vi "Control - Direct Injection.vi"(0 "Fuel Desired [mg/cyc]":sgl, 5 "MEP Desired [bar]":sgl, 11 "Control Inputs":T3={"Engine Speed [RPM]"=0.0, "Engine Status"=enum."STALLED", "Load Control \nMode"=enum."Max Speed Governor", "dt(s)"=0.0, "Number of Cylinders"=0, "Engine Displacement [cc]"=0.0, "StoichAFR"=0.0, "Q.LHV Fuel [kJ/kg]"=0.0, "BattV PSU [V]"=0.0, "12V PSU [V]"=0.0, "5V PSU [V]"=0.0, "Pedal Position [%]"=0.0, "Oil Pressure [kPa]"=0.0, "Oil Temp [C]"=0.0, "Oil Level [%]"=0.0, "Engine Coolant Temp (ECT) [C]"=0.0, "Engine Coolant Pressure [kPa]"=0.0, "Rail Pressure [bar]"=0.0, "Fuel Pressure [kPa]"=0.0, "Fuel Temp [C]"=0.0, "Vacuum Pressure [kPa]"=0.0, "Throttle Position [%]"=0.0, "Cam1 Advance [CAD]"=0.0, "Cam2 Advance [CAD]"=0.0, "Cam3 Advance [CAD]"=0.0, "Cam4 Advance [CAD]"=0.0, "CA50 Control Output [CAD]"=[], "CA50 Control Output Valid"=[], "Intake Air Temp (IAT) [C]"=0.0, "Barometric Air Pressure [kPa]"=0.0, "Intake Air Rel. Humidity [%]"=0.0, "Mass Air Flow (MAF) [kg/hr]"=0.0, "Turbo Inlet Air Pressure [kPa]"=0.0, "Turbo Inlet Air Temp [C]"=0.0, "Turbo Outlet Air Pressure [kPa]"=0.0, "Turbo Outlet Air Temp [C]"=0.0, "CAC Outlet Pressure [kPa]"=0.0, "CAC Outlet Temp [C]"=0.0, "Intake Manifold Pressure (MAP) [kPa]"=0.0, "Intake Manifold Temp (MAT) [C]"=0.0, "Exhaust Manifold Pressure [kPa]"=0.0, "Exhaust Manifold Temp [C]"=0.0, "HighP EGR Cooler Outlet Pressure [kPa]"=0.0, "HighP EGR Cooler Outlet Temp [C]"=0.0, "HighP EGR Differential Pressure [kPa]"=0.0, "HighP EGR Valve Position [%]"=0.0, "Turbo Outlet Exhaust Pressure [kPa]"=0.0, "Turbo Outlet Exhaust Temp [C]"=0.0, "VGT Position 1 [%]"=0.0, "VGT Position 2 [%]"=0.0, "Turbo Speed 1 [RPM]"=0.0, "Turbo Speed 2 [RPM]"=0.0, "LowP EGR Differential Pressure [kPa]"=0.0, "LowP EGR Valve Position [%]"=0.0, "UEGO1Lambda"=0.0, "UEGO1_Hot"=FALSE, "UEGO2Lambda"=0.0, "UEGO2_Hot"=FALSE, "Knock Intensity"=[], "Knock"=[]} {"Knock Intensity" format="%.2f"; "CA50 Control Output [CAD]" format="%.2f"; "Exhaust Manifold Temp [C]" format="%#_6f"; "UEGO2Lambda" format="%.2f"; "Intake Manifold Temp (MAT) [C]" format="%#_6f"; "UEGO1Lambda" format="%.2f"}) -> (4 "DI Quantities Desired [mg/inj]":T2[](array[typedef]), 8 "DI Timings Desired [DBTDC]":T1[](array[typedef]))   [LabVIEW 2015, in "ECS-RT.lvlib"]
uses:
  ECS-RT.lvlib
  Typedefs/Control Inputs/Control Inputs.ctl
  Typedefs/EPT/Engine Status.ctl
  Typedefs/MISC/Load Control Mode.ctl
  Typedefs/Control Outputs/Injection Quantity.ctl
  Typedefs/Control Outputs/Injection Timing.ctl
  ECS-Shared.lvlib
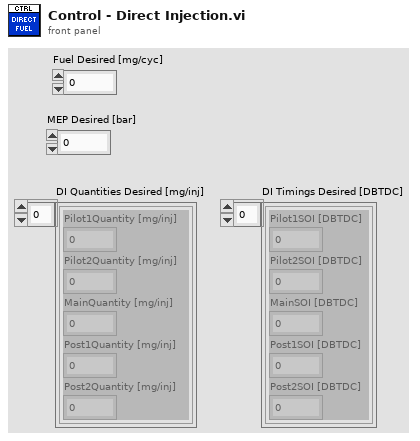
[diagram p1: front panel]
types:
  T1 = typedef "ECS-Shared.lvlib/Injection Timing.ctl" = cluster{"Pilot1SOI [DBTDC]":sgl, "Pilot2SOI [DBTDC]":sgl, "MainSOI [DBTDC]":sgl, "Post1SOI [DBTDC]":sgl, "Post2SOI [DBTDC]":sgl}
  T2 = typedef "ECS-Shared.lvlib/Injection Quantity.ctl" = cluster{"Pilot1Quantity [mg/inj]":sgl, "Pilot2Quantity [mg/inj]":sgl, "MainQuantity [mg/inj]":sgl, "Post1Quantity [mg/inj]":sgl, "Post2Quantity [mg/inj]":sgl}
  T3 = typedef "ECS-Shared.lvlib/Control Inputs.ctl" = cluster{"Engine Speed [RPM]":sgl, "Engine Status":T4, "Load Control \nMode":T5, "dt(s)":sgl, "Number of Cylinders":u8, "Engine Displacement [cc]":sgl, "StoichAFR":sgl, "Q.LHV Fuel [kJ/kg]":sgl, "BattV PSU [V]":sgl, "12V PSU [V]":sgl, "5V PSU [V]":sgl, "Pedal Position [%]":sgl, "Oil Pressure [kPa]":sgl, "Oil Temp [C]":sgl, "Oil Level [%]":sgl, "Engine Coolant Temp (ECT) [C]":sgl, "Engine Coolant Pressure [kPa]":sgl, "Rail Pressure [bar]":sgl, "Fuel Pressure [kPa]":sgl, "Fuel Temp [C]":sgl, "Vacuum Pressure [kPa]":sgl, "Throttle Position [%]":sgl, "Cam1 Advance [CAD]":sgl, "Cam2 Advance [CAD]":sgl, "Cam3 Advance [CAD]":sgl, "Cam4 Advance [CAD]":sgl, "CA50 Control Output [CAD]":sgl[], "CA50 Control Output Valid":bool[], "Intake Air Temp (IAT) [C]":sgl, "Barometric Air Pressure [kPa]":sgl, "Intake Air Rel. Humidity [%]":sgl, "Mass Air Flow (MAF) [kg/hr]":sgl, "Turbo Inlet Air Pressure [kPa]":sgl, "Turbo Inlet Air Temp [C]":sgl, "Turbo Outlet Air Pressure [kPa]":sgl, "Turbo Outlet Air Temp [C]":sgl, "CAC Outlet Pressure [kPa]":sgl, "CAC Outlet Temp [C]":sgl, "Intake Manifold Pressure (MAP) [kPa]":sgl, "Intake Manifold Temp (MAT) [C]":sgl, "Exhaust Manifold Pressure [kPa]":sgl, "Exhaust Manifold Temp [C]":sgl, "HighP EGR Cooler Outlet Pressure [kPa]":sgl, "HighP EGR Cooler Outlet Temp [C]":sgl, "HighP EGR Differential Pressure [kPa]":sgl, "HighP EGR Valve Position [%]":sgl, "Turbo Outlet Exhaust Pressure [kPa]":sgl, "Turbo Outlet Exhaust Temp [C]":sgl, "VGT Position 1 [%]":sgl, "VGT Position 2 [%]":sgl, "Turbo Speed 1 [RPM]":sgl, "Turbo Speed 2 [RPM]":sgl, "LowP EGR Differential Pressure [kPa]":sgl, "LowP EGR Valve Position [%]":sgl, "UEGO1Lambda":sgl, "UEGO1_Hot":bool, "UEGO2Lambda":sgl, "UEGO2_Hot":bool, "Knock Intensity":sgl[], "Knock":bool[]}
  T4 = typedef "ECS-Shared.lvlib/Engine Status.ctl" = enum16{"OFF", "STALLED", "CRANKING", "RUNNING", "ACCEL", "DECEL", "SAFE"}
  T5 = typedef "ECS-Shared.lvlib/Load Control Mode.ctl" = enum16{"No Governor", "Min Speed Governor", "Max Speed Governor"}
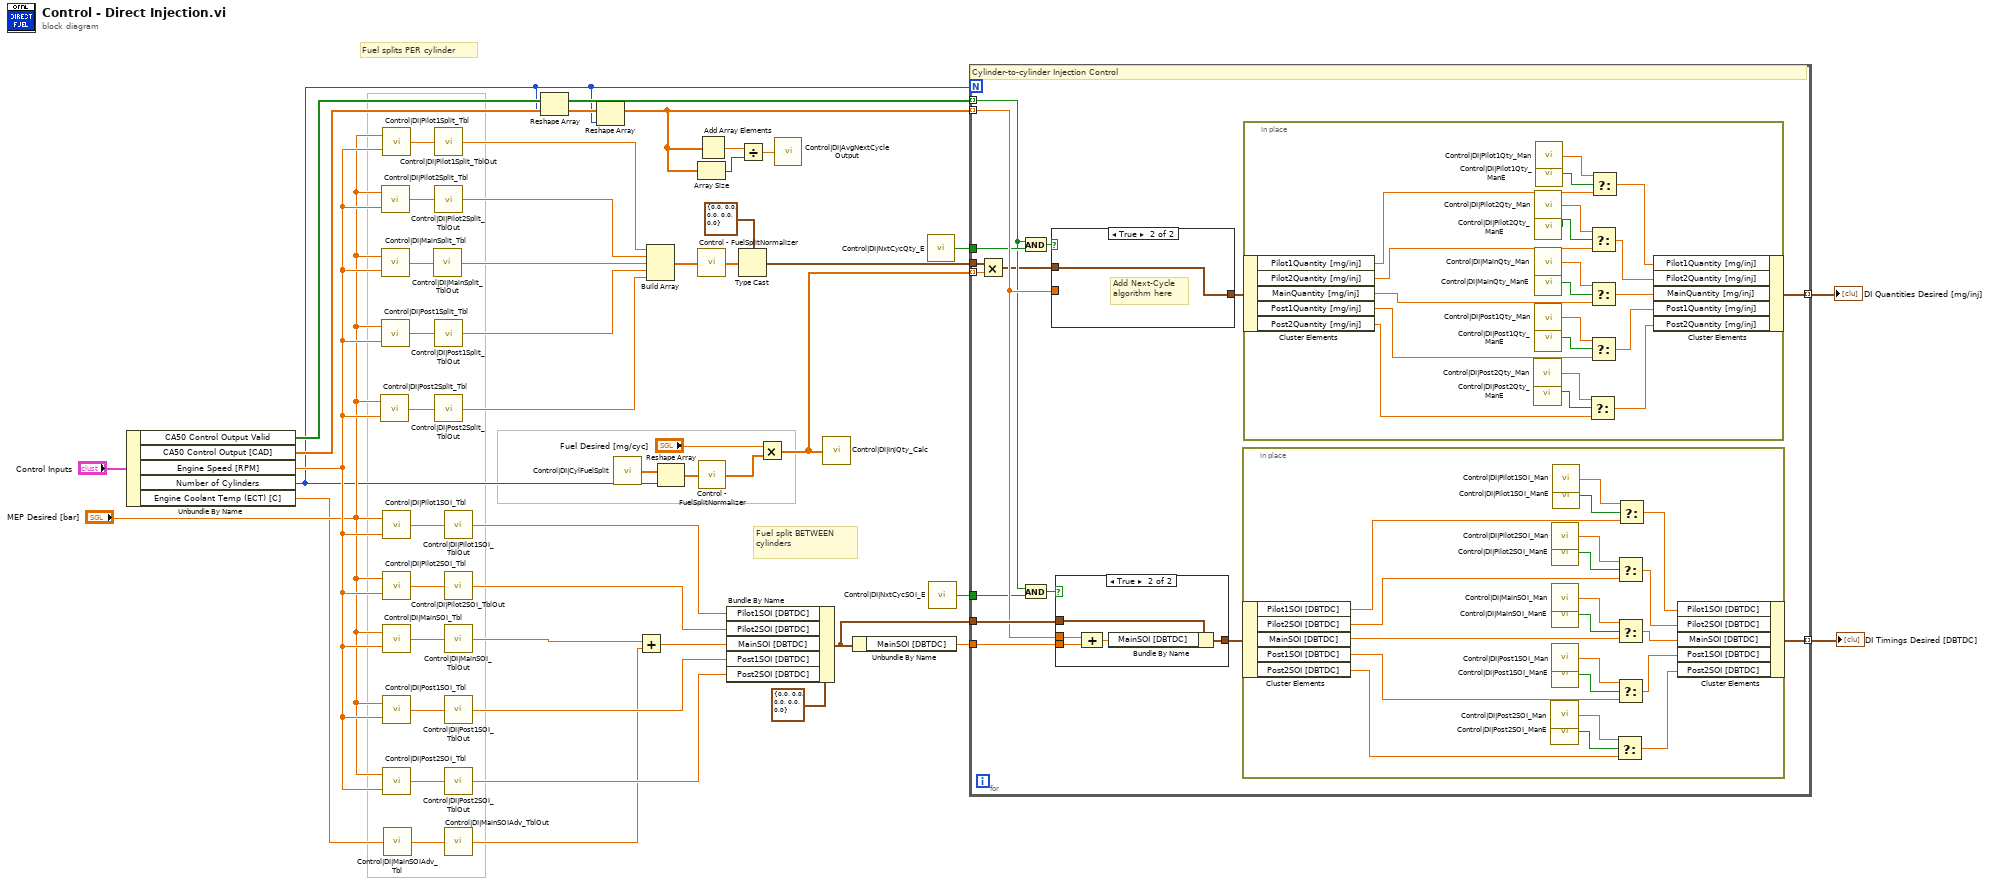
[diagram p0: block diagram]
diagram:
  # "Fuel split BETWEEN cylinders"
  # "Fuel splits PER cylinder"
  n1 = Unbundle By Name("Control Inputs") -> ("CA50 Control Output Valid"=w4:bool[], "CA50 Control Output [CAD]"=w5:sgl[], "Engine Speed [RPM]"=w20:sgl, "Number of Cylinders"=w1:u8, "Engine Coolant Temp (ECT) [C]"=w11:sgl)
  n2 = call "Control|DI|Post2Split_Tbl"("Y Index"=w20, "X Index"="MEP Desired [bar]") -> ("Z"=w29:sgl)
  n3 = call "Control|DI|Pilot2Split_Tbl"("Y Index"=w20, "X Index"="MEP Desired [bar]") -> ("Z"=w32:sgl)
  n4 = call "Control|DI|MainSplit_Tbl"("Y Index"=w20, "X Index"="MEP Desired [bar]") -> ("Z"=w31:sgl)
  n5 = call "Control|DI|Post1Split_Tbl"("Y Index"=w20, "X Index"="MEP Desired [bar]") -> ("Z"=w30:sgl)
  n6 = call "Control|DI|Pilot1Split_Tbl"("Y Index"=w20, "X Index"="MEP Desired [bar]") -> ("Z"=w33:sgl)
  n7 = call "Control|DI|Pilot1SOI_Tbl"("Y Index"=w20, "X Index"="MEP Desired [bar]") -> ("Z"=w40:sgl)
  n8 = call "Control|DI|Pilot2SOI_Tbl"("Y Index"=w20, "X Index"="MEP Desired [bar]") -> ("Z"=w39:sgl)
  n9 = call "Control|DI|MainSOI_Tbl"("Y Index"=w20, "X Index"="MEP Desired [bar]") -> ("Z"=w17:sgl)
  n10 = call "Control|DI|Post1SOI_Tbl"("Y Index"=w20, "X Index"="MEP Desired [bar]") -> ("Z"=w38:sgl)
  n11 = call "Control|DI|Post2SOI_Tbl"("Y Index"=w20, "X Index"="MEP Desired [bar]") -> ("Z"=w37:sgl)
  n12 = call "Control|DI|MainSOIAdv_Tbl"("X Index"=w11) -> ("Y"=w15:sgl)
  n13 = call "Control|DI|MainSplit_TblOut"("Value"=w31) -> ()
  n14 = call "Control|DI|Pilot1Split_TblOut"("Value"=w33) -> ()
  n15 = call "Control|DI|Pilot2Split_TblOut"("Value"=w32) -> ()
  n16 = call "Control|DI|Post1Split_TblOut"("Value"=w30) -> ()
  n17 = call "Control|DI|Post2Split_TblOut"("Value"=w29) -> ()
  n18 = call "Control|DI|Pilot1SOI_TblOut"("Value"=w40) -> ()
  n19 = call "Control|DI|Pilot2SOI_TblOut"("Value"=w39) -> ()
  n20 = call "Control|DI|MainSOI_TblOut"("Value"=w17) -> ()
  n21 = call "Control|DI|Post1SOI_TblOut"("Value"=w38) -> ()
  n22 = call "Control|DI|Post2SOI_TblOut"("Value"=w37) -> ()
  n23 = call "Control|DI|MainSOIAdv_TblOut"("Value"=w15) -> ()
  n24 = Reshape Array(w4, w1) -> (w2:bool[])
  n25 = Reshape Array(w5, w1) -> (w3:sgl[])
  n26 = call "Control|DI|CylFuelSplit"() -> ("Value"=w10:sgl[])
  n27 = Add(x=w17, y=w15) -> (x+y=w16:sgl)
  n28 = Build Array(w33, w32, w31, w30, w29) -> (w28:sgl[])
  n29 = Reshape Array(w10, w1) -> (w9:sgl[])
  n30 = Array Size(array=w3) -> (size(s)=w26:i32)
  n31 = call "Control - FuelSplitNormalizer.vi"("Fuel Splits []"=w28) -> ("Normalized Fuel Splits [Frac]"=w7:sgl[])  [unwired: 14 in]
  n32 = call "Control - FuelSplitNormalizer.vi"("Fuel Splits []"=w9) -> ("Normalized Fuel Splits [Frac]"=w14:sgl[])  [unwired: 14 in]
  n33 = Add Array Elements(numeric array=w3) -> (sum=w27:sgl)
  n34 = Bundle By Name(cluster=T1 {"Pilot1SOI [DBTDC]"=0.0, "Pilot2SOI [DBTDC]"=0.0, "MainSOI [DBTDC]"=0.0, "Post1SOI [DBTDC]"=0.0, "Post2SOI [DBTDC]"=0.0} ("FuelTiming [DBTDC] 2"), "Pilot1SOI [DBTDC]"=w40, "Pilot2SOI [DBTDC]"=w39, "MainSOI [DBTDC]"=w16, "Post1SOI [DBTDC]"=w38, "Post2SOI [DBTDC]"=w37) -> (w36:T1)
  n35 = Type Cast(type=T2 {"Pilot1Quantity [mg/inj]"=0.0, "Pilot2Quantity [mg/inj]"=0.0, "MainQuantity [mg/inj]"=0.0, "Post1Quantity [mg/inj]"=0.0, "Post2Quantity [mg/inj]"=0.0} ("Injection Quantity [mg/inj]"), x=w7) -> (*(type *) &x=w6:T2)
  n36 = Divide(x=w27, y=w26) -> (x/y=w25:sgl)
  n37 = Multiply(x="Fuel Desired [mg/cyc]", y=w14) -> (x*y=w13:sgl[])
  n38 = call "Control|DI|AvgNextCycleOutput"("Value"=w25) -> ()
  n39 = call "Control|DI|InjQty_Calc"("Value"=w13) -> ()
  n40 = Unbundle By Name(w36) -> ("MainSOI [DBTDC]"=w23:sgl)
  n41 = call "Control|DI|NxtCycQty_E"() -> ("Value"=w21:bool)
  n42 = call "Control|DI|NxtCycSOI_E"() -> ("Value"=w24:bool)
  n43 = for {
    N: w1 -> [_]
    tunnel: [w53] -> w34 mode=indexing
    tunnel: w23 -> [w49]
    tunnel: w36 -> [w55]
    tunnel: w24 -> [w44]
    tunnel: [w51] -> w22 mode=indexing
    tunnel: w2 -> [w45] mode=indexing
    tunnel: w3 -> [w48] mode=indexing
    tunnel: w21 -> [w46]
    tunnel: w6 -> [w42]
    tunnel: w13 -> [w43] mode=indexing
    # "Cylinder-to-cylinder Injection Control"
    n44 = Multiply(x=w42, y=w43) -> (x*y=w41:T2)
    n45 = And(x=w45, y=w46) -> (x .and. y?=w47:bool)
    n46 = And(x=w45, y=w44) -> (x .and. y?=w52:bool)
    n47 = case shown="True" w47 {
      tunnel: w48 -> [_ _]
      tunnel: [w56 w57] -> w50
      tunnel: w41 -> [w56 w57]
      frame False {
      }
      frame True {
        # "Add Next-Cycle\nalgorithm here"
      }
    }
    n48 = case shown="True" w52 {
      tunnel: [w98 w102] -> w54
      tunnel: w55 -> [w98 w99]
      tunnel: w49 -> [_ w101]
      tunnel: w48 -> [_ w100]
      frame False {
      }
      frame True {
        n49 = Compound Arithmetic op=ADD(w100, w101) -> (w103:sgl)
        n50 = Bundle By Name(cluster=w99, "MainSOI [DBTDC]"=w103) -> (w102:T1)
      }
    }
    n51 = in-place {
      n52 = in-place-cluster #1(w54) -> ("Pilot1SOI [DBTDC]"=w87:sgl, "Pilot2SOI [DBTDC]"=w86:sgl, "MainSOI [DBTDC]"=w85:sgl, "Post1SOI [DBTDC]"=w84:sgl, "Post2SOI [DBTDC]"=w83:sgl)
      n53 = call "Control|DI|Post2SOI_Man"() -> ("Value"=w96:sgl)
      n54 = call "Control|DI|Post2SOI_ManE"() -> ("Value"=w97:bool)
      n55 = call "Control|DI|Pilot2SOI_Man"() -> ("Value"=w92:sgl)
      n56 = call "Control|DI|Pilot2SOI_ManE"() -> ("Value"=w93:bool)
      n57 = call "Control|DI|MainSOI_Man"() -> ("Value"=w88:sgl)
      n58 = call "Control|DI|MainSOI_ManE"() -> ("Value"=w89:bool)
      n59 = call "Control|DI|Post1SOI_Man"() -> ("Value"=w94:sgl)
      n60 = call "Control|DI|Post1SOI_ManE"() -> ("Value"=w95:bool)
      n61 = call "Control|DI|Pilot1SOI_Man"() -> ("Value"=w90:sgl)
      n62 = call "Control|DI|Pilot1SOI_ManE"() -> ("Value"=w91:bool)
      n63 = Select(t=w96, s=w97, f=w83) -> (s? t:f=w78:sgl)
      n64 = Select(t=w92, s=w93, f=w86) -> (s? t:f=w81:sgl)
      n65 = Select(t=w88, s=w89, f=w85) -> (s? t:f=w80:sgl)
      n66 = Select(t=w94, s=w95, f=w84) -> (s? t:f=w79:sgl)
      n67 = Select(t=w90, s=w91, f=w87) -> (s? t:f=w82:sgl)
      n68 = in-place-cluster #1("Pilot1SOI [DBTDC]"=w82, "Pilot2SOI [DBTDC]"=w81, "MainSOI [DBTDC]"=w80, "Post1SOI [DBTDC]"=w79, "Post2SOI [DBTDC]"=w78) -> (w53:T1)
    }
    n69 = in-place {
      n70 = in-place-cluster #2(w50) -> ("Pilot1Quantity [mg/inj]"=w62:sgl, "Pilot2Quantity [mg/inj]"=w61:sgl, "MainQuantity [mg/inj]"=w60:sgl, "Post1Quantity [mg/inj]"=w59:sgl, "Post2Quantity [mg/inj]"=w58:sgl)
      n71 = call "Control|DI|Post2Qty_Man"() -> ("Value"=w69:sgl)
      n72 = call "Control|DI|Post2Qty_ManE"() -> ("Value"=w68:bool)
      n73 = call "Control|DI|Pilot2Qty_Man"() -> ("Value"=w74:sgl)
      n74 = call "Control|DI|Pilot2Qty_ManE"() -> ("Value"=w75:bool)
      n75 = call "Control|DI|MainQty_Man"() -> ("Value"=w72:sgl)
      n76 = call "Control|DI|MainQty_ManE"() -> ("Value"=w73:bool)
      n77 = call "Control|DI|Post1Qty_Man"() -> ("Value"=w71:sgl)
      n78 = call "Control|DI|Post1Qty_ManE"() -> ("Value"=w70:bool)
      n79 = call "Control|DI|Pilot1Qty_Man"() -> ("Value"=w76:sgl)
      n80 = call "Control|DI|Pilot1Qty_ManE"() -> ("Value"=w77:bool)
      n81 = Select(t=w69, s=w68, f=w58) -> (s? t:f=w63:sgl)
      n82 = Select(t=w74, s=w75, f=w61) -> (s? t:f=w66:sgl)
      n83 = Select(t=w72, s=w73, f=w60) -> (s? t:f=w65:sgl)
      n84 = Select(t=w71, s=w70, f=w59) -> (s? t:f=w64:sgl)
      n85 = Select(t=w76, s=w77, f=w62) -> (s? t:f=w67:sgl)
      n86 = in-place-cluster #2("Pilot1Quantity [mg/inj]"=w67, "Pilot2Quantity [mg/inj]"=w66, "MainQuantity [mg/inj]"=w65, "Post1Quantity [mg/inj]"=w64, "Post2Quantity [mg/inj]"=w63) -> (w51:T2)
    }
  }
  "DI Quantities Desired [mg/inj]" <- w22
  "DI Timings Desired [DBTDC]" <- w34
